vi "svl_Check Data Valid [Level] [Resampled].vi"(0 "even angle signal":T5 {"even angle signal" format="%.2f"; "dr" format="%.2f"; "r0" format="%.2f"}, 1 "exponential mode":enum16{"Slow", "Fast", "Impulse", "Custom"}(ring)=enum."Fast", 2 "time constant [ms]":dbl=125.0 format="%.2f", 5 "even angle channel info":T1={"channel name"="", "description"="", " channel info"={"sensor sensitivity"=1000.0, "engineering units"=1, "dB reference"=1.0, "custom label"="EU", "weighting filter"=0, "pregain"=0.0}} {"channel info"."pregain" format="%.2f"; "channel info"."weighting filter" items=["Linear", "A-weighting", "B-weighting", "C-weighting", "ITU-R 468-4", "Dolby", "CCITT", "C-message", "Wb", "Wc", "Wd", "We", "Wf", "Wh", "Wj", "Wk", "Wm", "AES17 20 kHz lowpass", "AES17 40 kHz lowpass", "AES17 20 kHz highpass", "AES17 40 kHz highpass"]; "channel info"."dB reference" format="%^.1e"; "channel info"."engineering units" items=["custom..."=0, "V"=1, "A"=21, "C"=30, "pC"=31, "s"=32, "-"=29, "Pa"=2, "N"=20, "g"=3, "m/s^2"=4, "m/s"=5, "m"=6, "mm/s"=12, "mm"=13, "micron/s"=14, "micron"=15, "in/s^2"=7, "in/s"=8, "in"=9, "mil/s"=10, "mil"=11, "rad/s^2"=16, "rad/s"=17, "rad"=18, "deg/s^2"=26, "deg/s"=27, "deg"=28, "RPM"=22, "cycle/s^2"=23, "Hz"=24, "cycle"=25, "strain"=19]; "channel info"."sensor sensitivity" format="%#_5f"}, 7 "Level Analysis":T6(ring), 9 "restart averaging (F)":bool, 11 "error in (no error)":errorcluster, 12 "integration time [s]":dbl=1.0 format="%.2f", 13 "decimation factor":i32=1 min=1 step=1) -> (4 "dup even angle signal":T5 {"even angle signal" format="%.2f"; "dr" format="%.2f"; "r0" format="%.2f"}, 6 "dup even angle channel info":T1={"channel name"="", "description"="", " channel info"={"sensor sensitivity"=1000.0, "engineering units"=1, "dB reference"=1.0, "custom label"="EU", "weighting filter"=0, "pregain"=0.0}} {"channel info"."pregain" format="%.2f"; "channel info"."weighting filter" items=["Linear", "A-weighting", "B-weighting", "C-weighting", "ITU-R 468-4", "Dolby", "CCITT", "C-message", "Wb", "Wc", "Wd", "We", "Wf", "Wh", "Wj", "Wk", "Wm", "AES17 20 kHz lowpass", "AES17 40 kHz lowpass", "AES17 20 kHz highpass", "AES17 40 kHz highpass"]; "channel info"."dB reference" format="%^.1e"; "channel info"."engineering units" items=["custom..."=0, "V"=1, "A"=21, "C"=30, "pC"=31, "s"=32, "-"=29, "Pa"=2, "N"=20, "g"=3, "m/s^2"=4, "m/s"=5, "m"=6, "mm/s"=12, "mm"=13, "micron/s"=14, "micron"=15, "in/s^2"=7, "in/s"=8, "in"=9, "mil/s"=10, "mil"=11, "rad/s^2"=16, "rad/s"=17, "rad"=18, "deg/s^2"=26, "deg/s"=27, "deg"=28, "RPM"=22, "cycle/s^2"=23, "Hz"=24, "cycle"=25, "strain"=19]; "channel info"."sensor sensitivity" format="%#_5f"}, 10 "processing state":T7(ring), 15 "error out":errorcluster)   [LabVIEW 2017]
uses:
  <vilib>/addons/_NISVFA/_Shared subVIs/Controls/svc_Resampled Channel Info.ctl
  <vilib>/addons/_NISVFA/_Shared subVIs/Controls/svc_Channel Info.ctl
  <vilib>/addons/_NISVFA/_Shared subVIs/Controls/svc_Engineering Units Text Ring.ctl
  <vilib>/addons/_NISVFA/_Shared subVIs/Controls/svc_Weighting Filter Text Ring.ctl
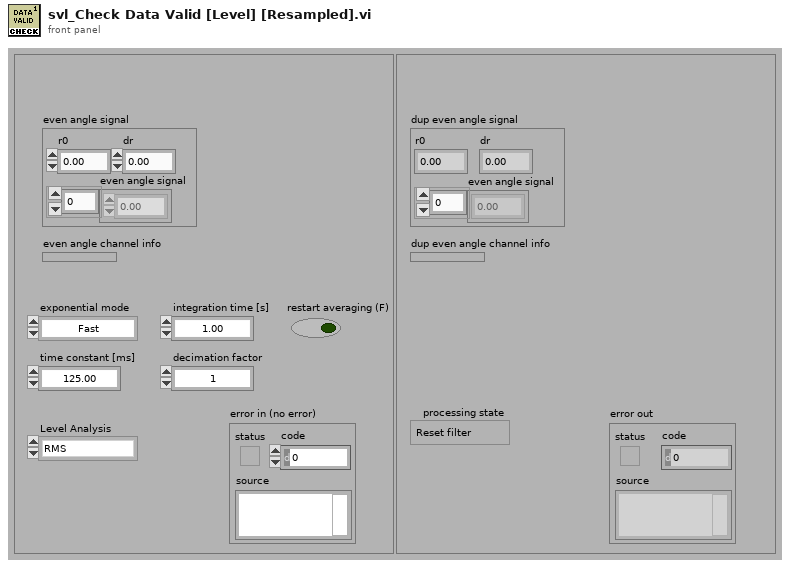
[diagram p1: front panel]
types:
  T1 = typedef "svc_Resampled Channel Info.ctl" = cluster{"channel name":string, "description":string, " channel info":T2}
  T2 = typedef "svc_Channel Info.ctl" = cluster{"sensor sensitivity":dbl, "engineering units":T3, "dB reference":dbl, "custom label":string, "weighting filter":T4, "pregain":dbl}
  T3 = typedef "svc_Engineering Units Text Ring.ctl" = u16
  T4 = typedef "svc_Weighting Filter Text Ring.ctl" = u16
  T5 = cluster{"r0":dbl, "dr":dbl, "even angle signal":dbl[]}
  T6 = enum16{"RMS", "Running RMS", "Exp avg  ", "Dec exp avg ", "Peak", "Crest"}
  T7 = enum16{"Reset filter", "Restart averaging", "Continue processing"}
  T8 = cluster{"ignore dt":bool, "ignore t0 continuity":bool, "ignore array length":bool, "ignore channel info":bool, "ignore channel name":bool}
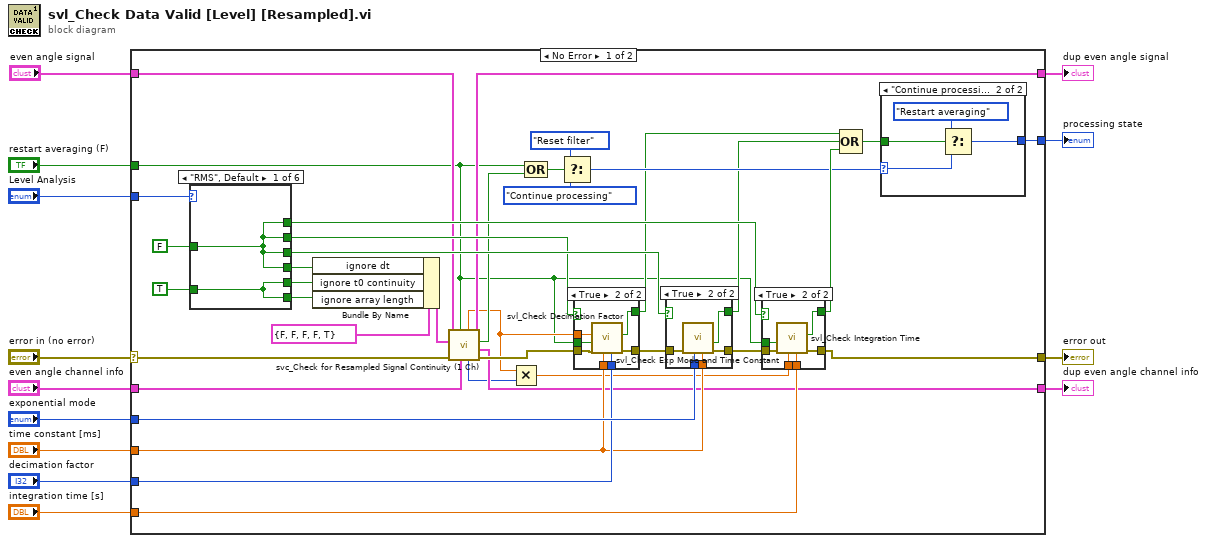
[diagram p0: block diagram]
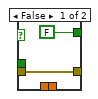
[diagram p3: hidden frame]
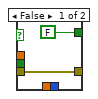
[diagram p4: hidden frame]
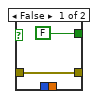
[diagram p5: hidden frame]
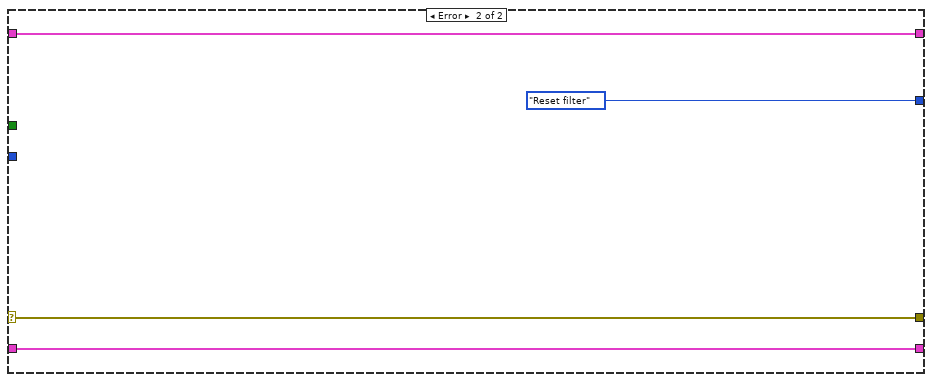
[diagram p11: hidden frame]
diagram:
  n1 = case shown="No Error" "error in (no error)" {
    selector: "error in (no error)" -> [w22 w96]
    tunnel: [w30 w96] -> w11
    tunnel: "restart averaging (F)" -> [w14 _]
    tunnel: "time constant [ms]" -> [w37 _]
    tunnel: [w43 T7."Reset filter" ("processing state")] -> w8
    tunnel: "Level Analysis" -> [w50 _]
    tunnel: "integration time [s]" -> [w49 _]
    tunnel: "decimation factor" -> [w48 _]
    tunnel: "exponential mode" -> [w51 _]
    tunnel: "even angle signal" -> [w21 w94]
    tunnel: [w20 w93] -> w3
    tunnel: [w19 w94] -> w2
    tunnel: "even angle channel info" -> [w18 w93]
    frame No Error {
      n2 = case shown="\"RMS\", Default" w50 {
        tunnel: [w82 w83 w85 w87 w90 w92] -> w42
        tunnel: [w82 w83 w86 w87 w90 w92] -> w41
        tunnel: [w82 w84 w86 w88 w90 w92] -> w40
        tunnel: [w81 w83 w85 w87 w89 w91] -> w24
        tunnel: [w81 w83 w86 w88 w89 w91] -> w34
        tunnel: [w82 w83 w86 w88 w89 w92] -> w33
        tunnel: FALSE -> [w82 w83 w86 w88 w90 w92]
        tunnel: TRUE -> [w81 w84 w85 w87 w89 w91]
        frame "RMS", Default {
        }
        frame "Running RMS" {
        }
        frame "Exp avg  " {
        }
        frame "Dec exp avg " {
        }
        frame "Peak" {
        }
        frame "Crest" {
        }
      }
      n3 = Bundle By Name(cluster=T8 {"ignore dt"=FALSE, "ignore t0 continuity"=FALSE, "ignore array length"=FALSE, "ignore channel info"=FALSE, "ignore channel name"=TRUE} ("parameter controls"), "ignore dt"=w33, "ignore t0 continuity"=w34, "ignore array length"=w24) -> (w35:T8)
      n4 = call <vilib>:"svc_Check for Resampled Signal Continuity (1 Ch).vi"("even angle channel info"=w18, "restart averaging (F)"=w14, "error in (no error)"=w22, "parameter controls"=w35, "even angle signal"=w21) -> ("error out"=w29:errorcluster, "dup even angle channel info"=w20:T1, "waveform parameter changed"=w23:bool, "dup even angle signal"=w19:T5, "array length"=w16:i32, "dt"=w17:dbl)  [unwired: 1 in]
      n5 = Multiply(x=w17, y=w16) -> (x*y=w15:dbl)
      n6 = Compound Arithmetic op=OR(w14, w23) -> (w38:bool)
      n7 = Select(t=T7."Reset filter" ("processing state"), s=w38, f=T7."Continue processing" ("processing state")) -> (s? t:f=w44:T7)
      n8 = case shown="True" w41 {
        tunnel: w29 -> [w66 w73]
        tunnel: [w66 w72] -> w32
        tunnel: w37 -> [_ w70]
        tunnel: w48 -> [_ w69]
        tunnel: [FALSE ("parameter has changed") w71] -> w27
        tunnel: w17 -> [_ w68]
        tunnel: w14 -> [_ w67]
        frame False {
        }
        frame True {
          n9 = call <vilib>:"svl_Check Decimation Factor.vi"("decimation factor"=w69, "time constant [ms]"=w70, "error in (no error)"=w73, "restart averaging (F)"=w67, "dt"=w68) -> ("error out"=w72:errorcluster, "parameter has changed"=w71:bool)  [unwired: 5 in]
        }
      }
      n10 = case shown="True" w42 {
        tunnel: w51 -> [_ w80]
        tunnel: w32 -> [w75 w76]
        tunnel: [w75 w79] -> w31
        tunnel: [FALSE w77] -> w28
        tunnel: w37 -> [_ w78]
        frame False {
        }
        frame True {
          n11 = call <vilib>:"svl_Check Exp Mode and Time Constant.vi"("time constant [ms]"=w78, "exponential mode"=w80, "error in (no error)"=w76) -> ("error out"=w79:errorcluster, "parameter has changed"=w77:bool)  [unwired: 7 in]
        }
      }
      n12 = case shown="True" w40 {
        tunnel: w31 -> [w58 w64]
        tunnel: [w58 w63] -> w30
        tunnel: w49 -> [_ w61]
        tunnel: [FALSE ("parameter has changed") w62] -> w47
        tunnel: w15 -> [_ w60]
        tunnel: w14 -> [_ w59]
        frame False {
        }
        frame True {
          n13 = call <vilib>:"svl_Check Integration Time.vi"("integration time"=w61, "acquisition period"=w60, "error in (no error)"=w64, "restart averaging (F)"=w59) -> ("error out"=w63:errorcluster, "parameter has changed"=w62:bool)  [unwired: 5 in, 1 out]
        }
      }
      n14 = Compound Arithmetic op=OR(w27, w28, w47) -> (w39:bool)
      n15 = case shown="\"Continue processing\"" w44 {
        selector: w44 -> [w52 w55]
        tunnel: w39 -> [_ w56]
        tunnel: [w52 w53] -> w43
        frame "Reset filter", Default {
        }
        frame "Continue processing" {
          n16 = Select(t=T7."Restart averaging" ("processing state"), s=w56, f=w55) -> (s? t:f=w53:T7)
        }
      }
    }
    frame Error {
      (unwired) TRUE ("t0 changed")
    }
  }
  "error out" <- w11
  "processing state" <- w8
  "dup even angle signal" <- w2
  "dup even angle channel info" <- w3
